vi "ejemplo.vi"() -> ()   [LabVIEW 2020]
uses:
  <vilib>/ErrorRing/Error Ring.xnode
panel:
  in  "Formato":string
  in  "Nombre del Archivo":string
  in  "Ruta de Almacenamiento":path
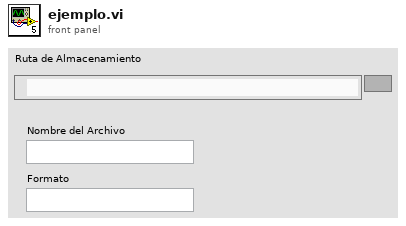
[diagram p1: front panel]
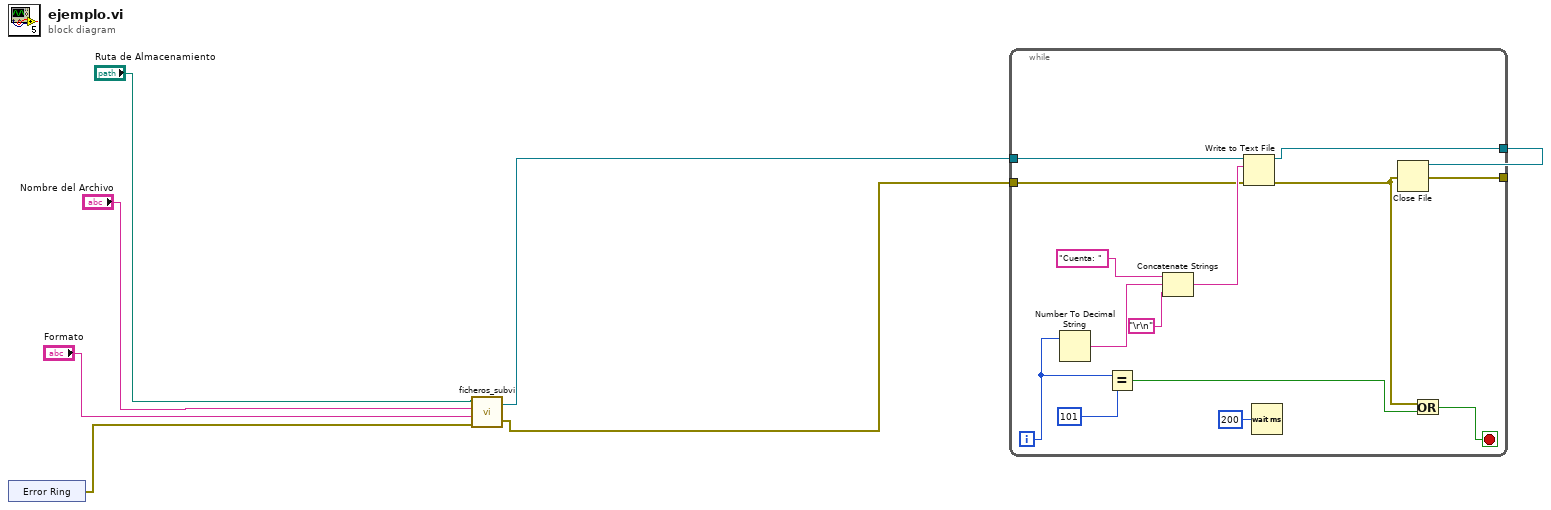
[diagram p0: block diagram]
diagram:
  n1 = xnode "Error Ring"() -> ("error out"=w3:errorcluster)
  n2 = call "ficheros_subvi.vi"("error in (no error)"=w3, "Formato"="Formato", "Nombre del Archivo"="Nombre del Archivo", "Ruta de Almacenamiento"="Ruta de Almacenamiento") -> ("error out"=w2:errorcluster, "Byte Stream File out"=w1:refnum<file>)
  n3 = while {
    tunnel: [w12] -> w8
    tunnel: [w11] -> w7
    tunnel: w2 -> [w10]
    tunnel: w1 -> [w9]
    i -> [w17]
    stop <- w15 stop-if-true
    n4 = Number To Decimal String(number=w17) -> (decimal integer string=w19:string)  [unwired: 1 in]
    n5 = Equal?(x=w17, y=101) -> (x = y?=w14:bool)
    n6 = Concatenate Strings("Cuenta: ", w19, "\r\n") -> (w13:string)
    n7 = Write to Text File(file (use dialog)=w9, text=w13, error in=w10) -> (refnum out=w12:refnum<file>, error out=w11:errorcluster)  [unwired: 1 in, 1 out]
    n8 = Wait (ms)(milliseconds to wait=u32 200) -> ()  [unwired: 1 out]
    n9 = Or(x=w11, y=w14) -> (x .or. y?=w15:bool)
  }
  n10 = Close File(refnum=w8, error in=w7) -> ()  [unwired: 2 out]
